vi "Not A Session - invalid session - returns true.vi"() -> ()   [LabVIEW 2017, in "unit_tests.lvlib"]
uses:
  unit_tests.lvlib
  libssh2/libssh2_init_default.vi
  libssh2/libssh2_session_init_ex.vi
  libssh2/libssh2.lvlib
  <vilib>/PNR/Transparent Assertions/Transparent Assertions/Transparent Assertions.lvlib
panel:
  out "error out":errorcluster
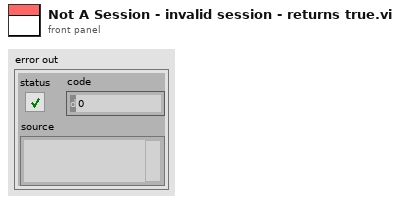
[diagram p1: front panel]
types:
  T1 = typedef "libssh2.lvlib/Session Refnum.ctl" = refnum<k1>
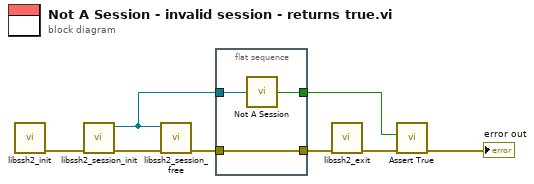
[diagram p0: block diagram]
diagram:
  n1 = call-poly "libssh2_init.vi"() -> ("error out"=w8:errorcluster)  [unwired: 11 in]
  n2 = call "libssh2_session_init.vi"("error in (no error)"=w8) -> ("error out"=w4:errorcluster, "session"=w3:T1)  [unwired: 9 in]
  n3 = call "libssh2_session_free.vi"("error in (no error)"=w4, "session"=w3) -> ("error out"=w2:errorcluster)  [unwired: 9 in]
  n4 = flat-sequence {
    tunnel: [w11] -> w5
    tunnel: w3 -> [w10]
    tunnel: w2 -> [w9]
    tunnel: [w9] -> w1
    frame #0 {
      n5 = call "Not A Session.vi"("session"=w10) -> ("Not a Session?"=w11:bool)
    }
  }
  n6 = call "libssh2_exit.vi"("error in (no error)"=w1) -> ("error out"=w6:errorcluster)  [unwired: 10 in]
  n7 = call <vilib>:"Assert True.vi"("error in (no error)"=w6, "Condition"=w5) -> ("error out"=→"error out":errorcluster)  [unwired: 9 in]
